vi "main.vi"() -> ()   [LabVIEW 2014]
panel:
  in  "stop":bool
  out "Error Out":errorcluster
  out "True: record":bool
  in  "Camera Type":string="Neo"
  in  "Schedule":cluster{"UTC ON hour":i32, "UTC OFF hour":i32}={"UTC ON hour"=22, "UTC OFF hour"=8}
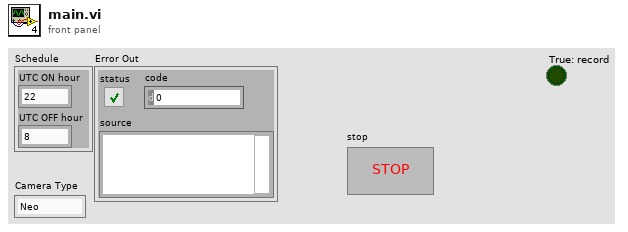
[diagram p1: front panel]
types:
  T1 = cluster{"AOIHeight":i64, "AOIWidth":i64, "AOIStride":i64, "ImageSizeBytes":i64, "Pixel Encoding":string}
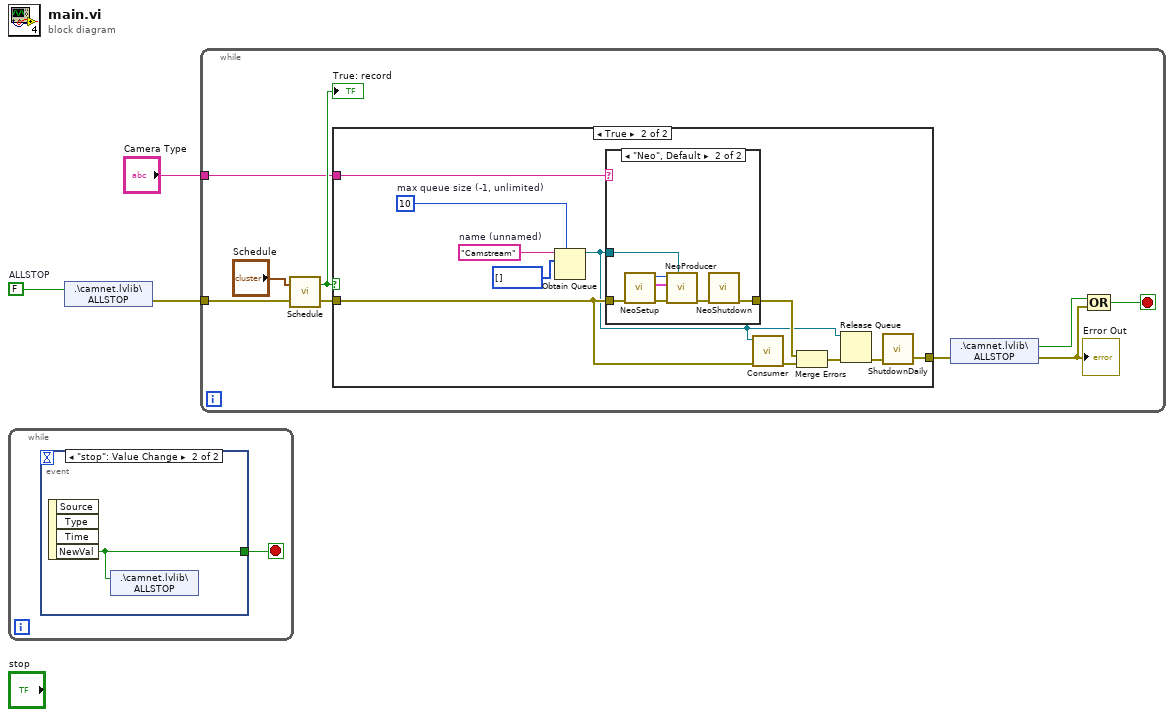
[diagram p0: block diagram]
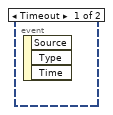
[diagram p2: hidden frame]
diagram:
  w1 = FALSE  # ALLSTOP
  n1 = while {
    stop <- w4 stop-if-true
    n2 = event shown="[1] \"stop\": Value Change" {
      selector: _ -> [_ _]
      dyn-events: _ -> [_ _]
      timeout: _ -> [_ _]
      tunnel: [_ w5] -> w4
      event Timeout {
        n3 = event-data() -> ()  [unwired: 1 in, 3 out]
      }
      event "stop": Value Change {
        n4 = event-data() -> ("NewVal"=w5:bool)  [unwired: 1 in, 3 out]
        n5 = shared-variable ".\\camnet.lvlib\\ALLSTOP"(w5) -> ()  [unwired: 1 in, 1 out]
      }
    }
  }
  n6 = shared-variable ".\\camnet.lvlib\\ALLSTOP"(w1) -> (error out=w2:errorcluster)  [unwired: 1 in]
  n7 = while {
    tunnel: "Camera Type" -> [w8]
    tunnel: w2 -> [w6]
    stop <- w14 stop-if-true
    n8 = call "Schedule.vi"("error in (no error)"=w6, "Schedule"="Schedule") -> ("error out"=w10:errorcluster, "True: record"=w12:bool)
    "True: record" <- w12
    n9 = case shown="True" w12 {
      tunnel: [w15 w24] -> w9
      tunnel: w10 -> [w15 w22]
      tunnel: w8 -> [_ w26]
      frame False {
      }
      frame True {
        w19 = 10  # max queue size (-1, unlimited)
        w21 = "Camstream"  # name (unnamed)
        n10 = Obtain Queue(max queue size (-1, unlimited)=w19, name (unnamed)=w21, element data type=u16[] []) -> (queue out=w16:refnum<queue>)  [unwired: 2 in, 2 out]
        n11 = case shown="\"Neo\", Default" w26 {
          tunnel: w22 -> [w27 w34]
          tunnel: [w27 w31] -> w25
          tunnel: w16 -> [_ w28]
          frame "Ultra" {
          }
          frame "Neo", Default {
            n12 = call "NeoSetup.vi"("Error In"=w34) -> ("ErrorOut"=w33:errorcluster, "NeoParam"=w30:T1, "Handle"=w29:i32)  [unwired: 4 in]
            n13 = call "NeoProducer.vi"("queue in"=w28, "Error In"=w33, "NeoParam 2"=w30, "Handle"=w29) -> ("Error Out"=w32:errorcluster)  [unwired: 7 in]
            n14 = call "NeoShutdown.vi"("Error In"=w32) -> ("ErrorOut"=w31:errorcluster)  [unwired: 6 in]
          }
        }
        n15 = call "Consumer.vi"("Error In"=w22, "queue in"=w16) -> ("ErrorOut"=w23:errorcluster)  [unwired: 5 in]
        n16 = Merge Errors(w25, w23) -> (w18:errorcluster)
        n17 = Release Queue(queue=w16, error in (no error)=w18) -> (error out=w17:errorcluster)  [unwired: 1 in, 2 out]
        n18 = call "ShutdownDaily.vi"("Error In"=w17) -> ("ErrorOut"=w24:errorcluster)  [unwired: 3 in]
      }
    }
    n19 = shared-variable ".\\camnet.lvlib\\ALLSTOP"(error in=w9) -> (w13:bool, error out=w7:errorcluster)
    "Error Out" <- w7
    n20 = Compound Arithmetic op=OR(w13, w7) -> (w14:bool)
  }
